vi "FFT_DAS_Header Columns for LogFile.vi"(8 "error in":errorcluster) -> (0 "error out":errorcluster, 2 "2D Header Columns":string[][](array[string]))   [LabVIEW 2010]
doc: "Simply acts as a compact constant for the column headers for the data log file.\nThis could be replaced later with a VI that reads a file to get the headers.\n\n2010_09\nMichael Ashe\nmichael.ashe@imaginatics.net\n(860) 664-8882"
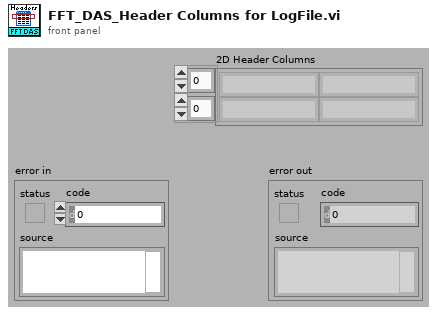
[diagram p1: front panel]
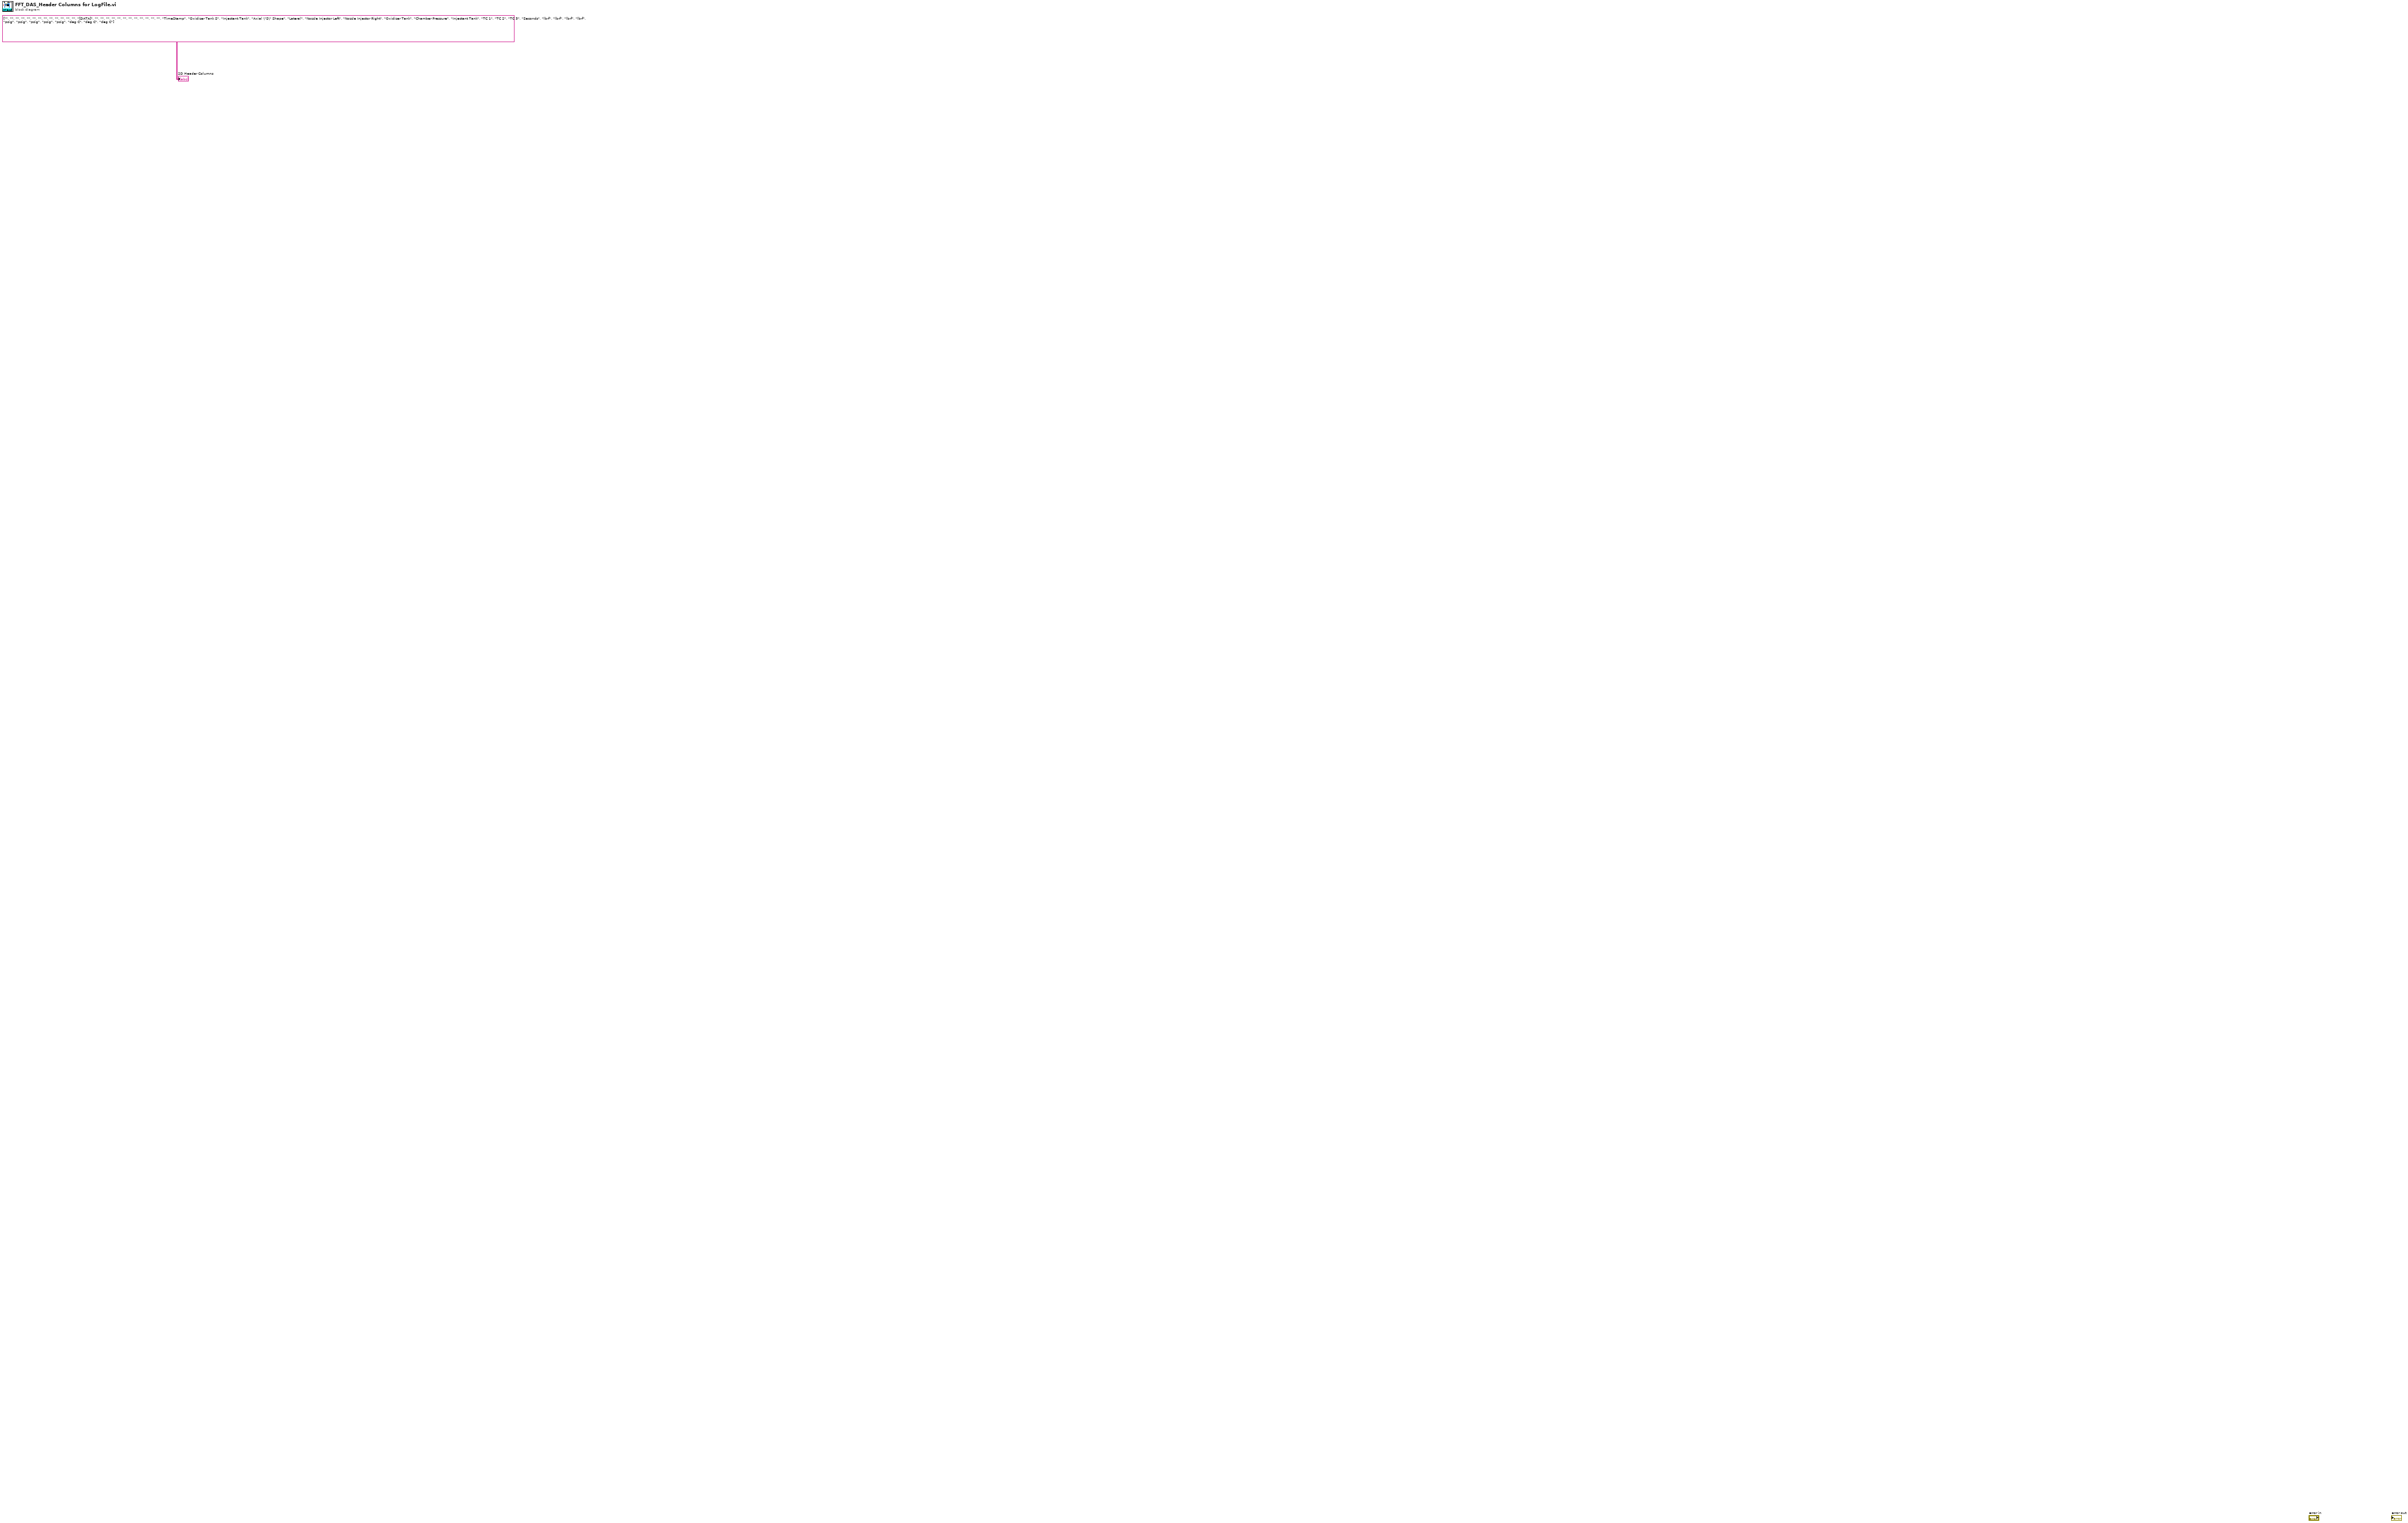
[diagram p0: block diagram]
diagram:
  "2D Header Columns" <- string[][] [["", "", "", "", "", "", "", "", "", "", "", "", ""], ["[DATA]", "", "", "", "", "", "", "", "", "", "", "", ""], ["TimeStamp", "Oxidizer Tank S", "Injectant Tank", "Axial \"S\" Shape", "Lateral", "Nozzle Injector Left", "Nozzle Injector Right", "Oxidizer Tank", "Chamber Pressure", "Injectant Tank", "TC 1", "TC 2", "TC 3"], ["Seconds", "lb-f", "lb-f", "lb-f", "lb-f", "psig", "psig", "psig", "psig", "psig", "deg C", "deg C", "deg C"]] ("1D data")
